vi "Read CVT.vi"(8 "error in (no error)":errorcluster, 11 "CVT in":refnum<class "CVT.lvclass">) -> (0 "error out":errorcluster, 2 "CVT":variant, 3 "CVT out":refnum<class "CVT.lvclass">)   [LabVIEW 2014, in "CVT.lvclass"]
uses:
  CVT.lvclass
  CVT.lvclass/CVT.ctl
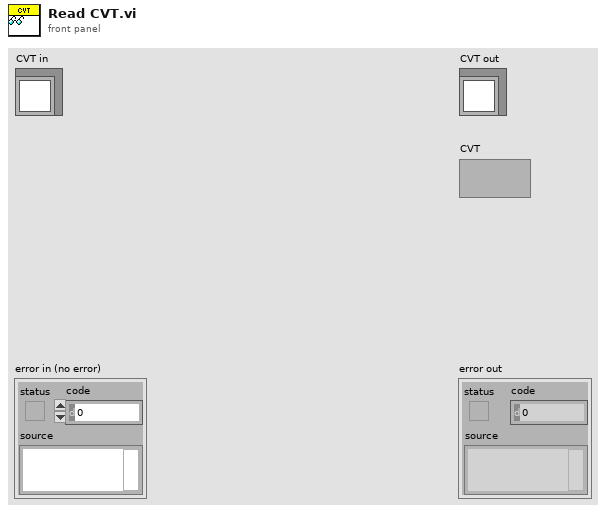
[diagram p1: front panel]
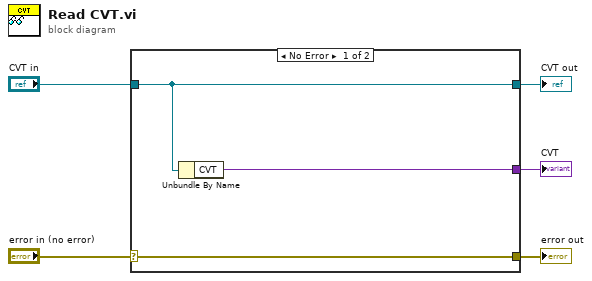
[diagram p0: block diagram]
diagram:
  n1 = case shown="No Error" "error in (no error)" {
    selector: "error in (no error)" -> [w8 w9]
    tunnel: [w8 w9] -> w4
    tunnel: [w7 w10] -> w2
    tunnel: "CVT in" -> [w7 w10]
    tunnel: [w6 _] -> w1
    frame No Error {
      n2 = Unbundle By Name(w7) -> ("CVT"=w6:variant)
    }
    frame Error {
    }
  }
  "error out" <- w4
  "CVT out" <- w2
  "CVT" <- w1
